vi "CALC_FUNC_TYPE.vi"(0 "VISA IN":refnum<visa-resource-name>, 1 "Function Type":string, 5 "error in":errorcluster, 7 "Channel":i32) -> (14 "VISA Out":refnum<visa-resource-name>, 19 "error out":errorcluster)   [LabVIEW 2018, in "PNA-X.lvlib"]
doc: "CALCulate<cnum>:FUNCtion:TYPE <char> \n1519\n\n(Read-Write) Sets statistic TYPE that you can then query using CALC:FUNCtion:DATA?. \nNote: In PNA releases 4.2 and prior, this command applied the statistic type to all measurements. \nNow, this command affects only the selected measurement on the specified channel. \nSee Critical Note \nParameters \n<cnum> Channel number of the measurement. There must be a selected measurement \non that channel. If unspecified, <cnum> is set to 1. \n<char> Choose from: \nPTPeak - the difference between the max and min data points on the trace. \nSTDEV - standard deviation of all data points on the trace \nMEAN - mean (average) of all data points on the trace \nMIN - lowest data point on the trace \nMAX - highest data point on the trace \nExamples CALC:FUNC:TYPE PTP \ncalculate2:function:type stdev \nQuery Syntax CALCulate<cnum>:FUNCtion:TYPE? \nReturn Type Character \nDefault PTPeak \n1520\n\nCalc:Limit Commands \nControls the limit segments used for pass / fail testing. \nClick on a blue keyword to view the command details. \nSee Also \nExample Programs \nLearn about Limit Lines \nSynchronizing the PNA and Controller \nSCPI Command Tree \nCritical Note: CALCulate commands act on the selected measurement. You can select one \nmeasurement for each channel using Calc:Par:Select"
uses:
  PNA-X.lvlib
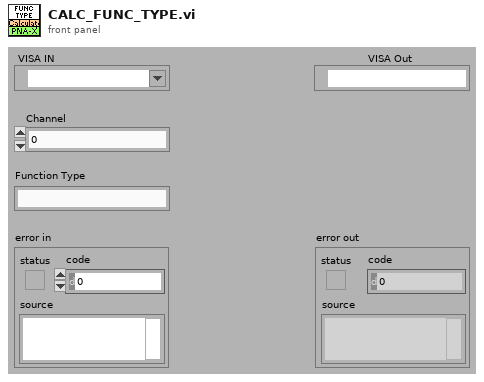
[diagram p1: front panel]
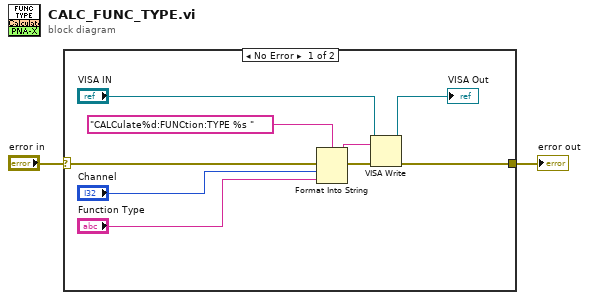
[diagram p0: block diagram]
diagram:
  n1 = case shown="No Error" "error in" {
    selector: "error in" -> [w11 w12]
    tunnel: [w6 w12] -> w1
    frame No Error {
      n2 = Format Into String(format string="CALCulate%d:FUNCtion:TYPE %s " ("Cmdline"), error in=w11, "Channel", "Function Type") -> (resulting string=w9:string, error out=w10:errorcluster)  [unwired: 1 in]
      n3 = VISA Write(VISA resource name="VISA IN", write buffer=w9, error in (no error)=w10) -> (VISA resource name out=→"VISA Out":refnum<visa-resource-name>, error out=w6:errorcluster)  [unwired: 1 out]
    }
    frame Error {
    }
  }
  "error out" <- w1
